vi "PWM User Variable FPGA Demo.vi"   [LabVIEW 2025]
uses:
  <vilib>/Platform/TimedLoop/XDataNode/timing_clust.ctl
  <vilib>/Platform/TimedLoop/XDataNode/nitl_modes.ctl
  <vilib>/Platform/TimedLoop/XDataNode/wakeup.ctl
  FPGA IP/Types/PWM.Measure.Digital.Settings.ctl
  FPGA IP/Types/PWM.Generate.Digital.Settings.ctl
  <vilib>/rvi/Emulation/niFpgaSctlEmulationGetInTimedLoop.vi
  <vilib>/rvi/Emulation/niFpgaEmulationReportErrorSimple.vi
  <vilib>/rvi/Emulation/niFpgaGetClockAttributes.vi
  <vilib>/rvi/Emulation/niFpgaCriticalErrorInLSC.vi
  <vilib>/rvi/eio/common/nirviEmuTemplateMethod_errors.vi
  <vilib>/platform/TimedLoop/XDataNode/XDataNode.xnode
  <vilib>/eio/EIONode/EIONode.xnode
  FPGA IP/Speciality FPGA IO.lvlib
  <vilib>/Platform/TimedLoop/XDataNode/XDNodeRunTimeDep.lvlib
types:
  T1 = typedef "XDNodeRunTimeDep.lvlib/timing_clust.ctl" = cluster{"Expected End [f-1]":u64, "Actual End [f-1]":u64, "Finished Late? [f-1]":bool, "Expected End [i-1]":u64, "Actual End [i-1]":u64, "Finished Late? [i-1]":bool, "Expected Start [i]":u64, "Actual Start [i]":u64, "Expected Start [f]":u64, "Actual Start [f]":u64, "Source Name":string, "Structure Name":string, "Period":i64, "Deadline":i64, "Offset":i64, "Start":i64, "Priority":i32, "Timeout":i32, "Mode":T2, "Wakeup Reason":T3, "Error":errorcluster, "Source Type":string, "Secondary Source Type":string, "Global End Time":u64, "Global Start Time":u64, "Frame Duration":u64, "Iteration Duration":u64, "Assigned CPU":i32, "I/O Scan Engine Mode":u32}
  T2 = typedef "XDNodeRunTimeDep.lvlib/nitl_modes.ctl" = enum32{"No Change", "Process missed periods, maintain original phase", "Discard missed periods, maintain original phase", "Process missed periods, ignore original phase", "Discard missed periods, ignore original phase"}
  T3 = typedef "XDNodeRunTimeDep.lvlib/wakeup.ctl" = enum32{"Normal", "Aborted", "Asynchronous wakeup", "Timing source error", "Timed loop error", "Timeout"}
  T4 = typedef "Speciality FPGA IO.lvlib/PWM.Generate.Digital.Settings.ctl" = cluster{"ACTIVE EDGE":bool, "ACTIVE TICKS":u32, "INACTIVE TICKS":u32}
  T5 = typedef "Speciality FPGA IO.lvlib/PWM.Measure.Digital.Settings.ctl" = cluster{"ACTIVE EDGE":bool, "TIMEOUT":u32}
  T6 = typedef "Speciality FPGA IO.lvlib/PWM.Measure.Digital.Measurement.ctl" = cluster{"ACTIVE TICKS":u32, "INACTIVE TICKS":u32, "ACQ TICKS":u32}
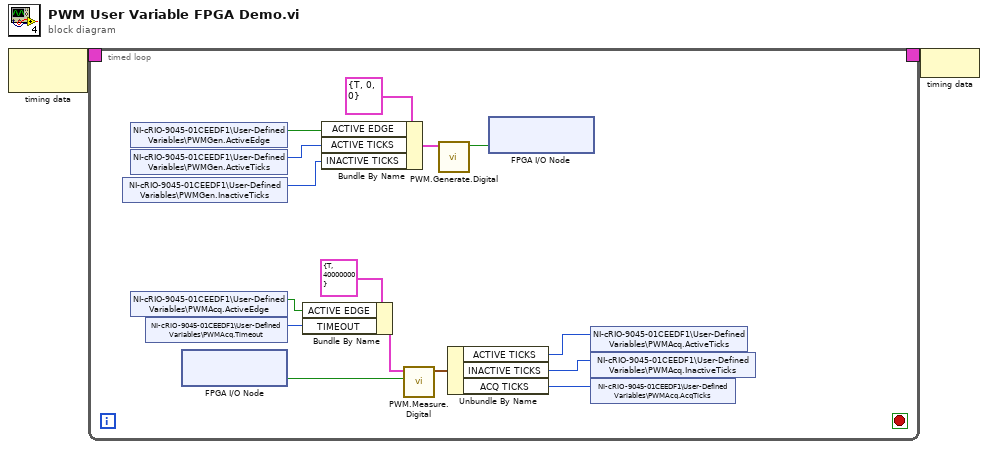
[diagram p0: block diagram]
diagram:
  n1 = node-c288() -> (w2:T1)  [unwired: 1 in]
  n2 = timed-loop {
    timing: w2 -> [_]
    timing-out: [_] -> w1
    stop <- _ stop-if-true
    n3 = shared-variable "NI-cRIO-9045-01CEEDF1\\User-Defined Variables\\PWMGen.InactiveTicks"() -> (w5:u32)  [unwired: 1 in, 1 out]
    n4 = shared-variable "NI-cRIO-9045-01CEEDF1\\User-Defined Variables\\PWMGen.ActiveEdge"() -> (w7:bool)  [unwired: 1 in, 1 out]
    n5 = shared-variable "NI-cRIO-9045-01CEEDF1\\User-Defined Variables\\PWMGen.ActiveTicks"() -> (w6:u32)  [unwired: 1 in, 1 out]
    n6 = shared-variable "NI-cRIO-9045-01CEEDF1\\User-Defined Variables\\PWMAcq.ActiveEdge"() -> (w4:bool)  [unwired: 1 in, 1 out]
    n7 = shared-variable "NI-cRIO-9045-01CEEDF1\\User-Defined Variables\\PWMAcq.Timeout"() -> (w3:u32)  [unwired: 1 in, 1 out]
    n8 = xnode "FPGA I/O Node"() -> ("Mod2/DIO3"=w16:bool)  [unwired: 1 in, 1 out]
    n9 = Bundle By Name(cluster=T5 {"ACTIVE EDGE"=TRUE, "TIMEOUT"=40000000} ("Mod2.Ch3.PWMIn.Settings"), "ACTIVE EDGE"=w4, "TIMEOUT"=w3) -> (w11:T5)
    n10 = Bundle By Name(cluster=T4 {"ACTIVE EDGE"=TRUE, "ACTIVE TICKS"=0, "INACTIVE TICKS"=0} ("Mod2.Ch4.PWMOut.Settings"), "ACTIVE EDGE"=w7, "ACTIVE TICKS"=w6, "INACTIVE TICKS"=w5) -> (w12:T4)
    n11 = call "PWM.Measure.Digital.vi"("State"=w16, "Settings"=w11) -> ("Measurement"=w13:T6)  [unwired: 8 in, 1 out]
    n12 = call "PWM.Generate.Digital.vi"("Settings"=w12) -> ("Output"=w17:bool)  [unwired: 10 in]
    n13 = Unbundle By Name(w13) -> ("ACTIVE TICKS"=w8:u32, "INACTIVE TICKS"=w9:u32, "ACQ TICKS"=w10:u32)
    n14 = xnode "FPGA I/O Node"("Mod2/DIO4"=w17) -> ()  [unwired: 1 in, 1 out]
    n15 = shared-variable "NI-cRIO-9045-01CEEDF1\\User-Defined Variables\\PWMAcq.ActiveTicks"(w8) -> ()  [unwired: 1 in, 1 out]
    n16 = shared-variable "NI-cRIO-9045-01CEEDF1\\User-Defined Variables\\PWMAcq.InactiveTicks"(w9) -> ()  [unwired: 1 in, 1 out]
    n17 = shared-variable "NI-cRIO-9045-01CEEDF1\\User-Defined Variables\\PWMAcq.AcqTicks"(w10) -> ()  [unwired: 1 in, 1 out]
  }
  n18 = node-c288(w1) -> ()
